vi "_TreeItem.Property.Set.Dictionary.Write.vi"(8 "error in (no error)":errorcluster, 11 "Dictionary":T1) -> (0 "error out":errorcluster, 3 "DictionaryProperty":refnum<k24>)   [LabVIEW 2017, in "Advanced System Definition.lvlib"]
uses:
  SysDef API/Advanced System Definition.lvlib
  _Types/Property.Dictionary.ctl
  NationalInstruments.VeriStand.SystemStorage
  _Types/Dictionary Item.ctl
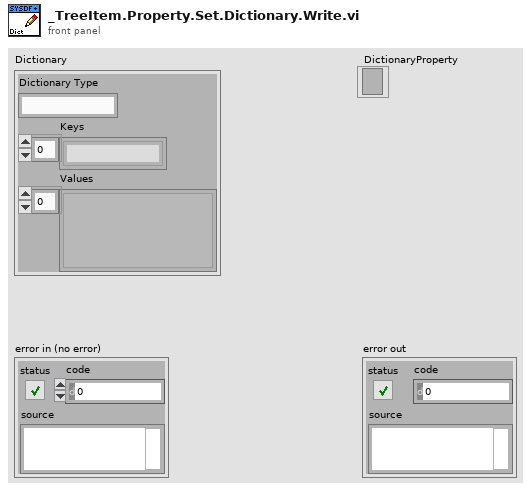
[diagram p1: front panel]
types:
  T1 = typedef "Advanced System Definition.lvlib/Property.Dictionary.ctl" = cluster{"Dictionary Type":string, "Keys":string[], "Values":variant[]}
  T2 = typedef "Advanced System Definition.lvlib/Dictionary Item.ctl" = cluster{"index":i32, "key":string, "value":variant}
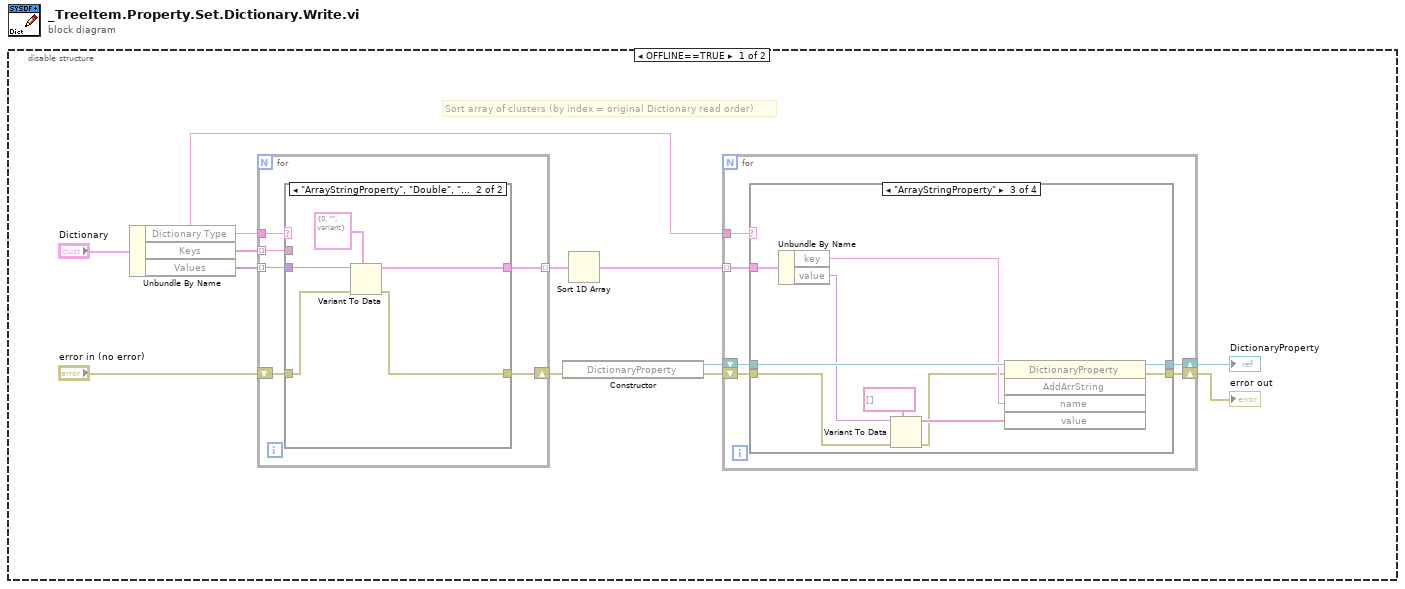
[diagram p0: block diagram]
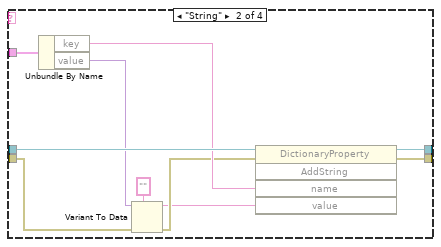
[diagram p3: hidden frame]
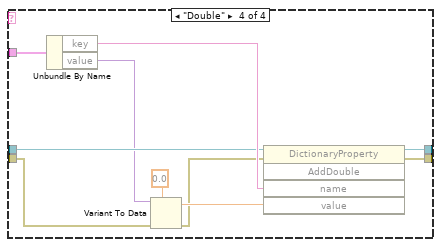
[diagram p4: hidden frame]
diagram:
  n1 = disable-structure shown="OFFLINE==TRUE" {
    frame condition #0 {
      # "Sort array of clusters (by index = original Dictionary read order)"
      n2 = Unbundle By Name("Dictionary") -> ("Dictionary Type"=w9:string, "Keys"=w10:string[], "Values"=w11:variant[])
      n3 = for {
        tunnel: w9 -> [w56]
        tunnel: w11 -> [w55] mode=indexing
        tunnel: w10 -> [w54] mode=indexing
        shift-right: [w52] -> w4
        shift-left: "error in (no error)" -> [w53]
        tunnel: [w51] -> w6 mode=indexing
        n4 = case shown="\"ArrayStringProperty\", \"Double\", \"String\"" w56 {
          tunnel: w54 -> [_ _]
          tunnel: w55 -> [_ w62]
          tunnel: w53 -> [w57 w61]
          tunnel: [w57 w60] -> w52
          tunnel: [_ w59] -> w51
          frame Default {
          }
          frame "ArrayStringProperty", "Double", "String" {
            n5 = Variant To Data(error in=w61, type=T2 {"index"=0, "key"="", "value"=variant} ("Dictionary Item"), Variant=w62) -> (data=w59:T2, error out=w60:errorcluster)
          }
        }
      }
      n6 = constructor class="DictionaryProperty"(error in=w4) -> (reference out=w2:refnum<k24>, error out=w3:errorcluster)  [unwired: 2 in, 1 out]
      n7 = Sort 1D Array(array=w6) -> (sorted array=w5:T2[])
      n8 = for {
        shift-right: [w17] -> w8
        shift-left: w2 -> [w18]
        tunnel: w9 -> [w16]
        shift-right: [w14] -> w7
        shift-left: w3 -> [w15]
        tunnel: w5 -> [w13] mode=indexing
        n9 = case shown="\"ArrayStringProperty\"" w16 {
          tunnel: w18 -> [w20 w30 w40 w46]
          tunnel: [w20 w29 w39 w50] -> w17
          tunnel: w15 -> [w19 w23 w32 w42]
          tunnel: [w19 w28 w38 w49] -> w14
          tunnel: w13 -> [_ w27 w36 w47]
          frame Default {
          }
          frame "String" {
            n10 = Unbundle By Name(w27) -> ("key"=w26:string, "value"=w24:variant)
            n11 = Variant To Data(error in=w23, type="", Variant=w24) -> (data=w21:string, error out=w22:errorcluster)
            n12 = invoke class="DictionaryProperty" method="AddString"(reference=w30, error in=w22, "name"=w26, "value"=w21) -> (reference out=w29:refnum<k24>, error out=w28:errorcluster)  [unwired: 1 in, 3 out]
          }
          frame "ArrayStringProperty" {
            n13 = Unbundle By Name(w36) -> ("key"=w37:string, "value"=w34:variant)
            n14 = Variant To Data(error in=w32, type=string[] [], Variant=w34) -> (data=w33:string[], error out=w31:errorcluster)
            n15 = invoke class="DictionaryProperty" method="AddArrString"(reference=w40, error in=w31, "name"=w37, "value"=w33) -> (reference out=w39:refnum<k24>, error out=w38:errorcluster)  [unwired: 1 in, 3 out]
          }
          frame "Double" {
            n16 = Unbundle By Name(w47) -> ("key"=w48:string, "value"=w44:variant)
            n17 = Variant To Data(error in=w42, type=0.0, Variant=w44) -> (data=w43:dbl, error out=w41:errorcluster)
            n18 = invoke class="DictionaryProperty" method="AddDouble"(reference=w46, error in=w41, "name"=w48, "value"=w43) -> (reference out=w50:refnum<k24>, error out=w49:errorcluster)  [unwired: 1 in, 3 out]
          }
        }
      }
      "error out" <- w7
      "DictionaryProperty" <- w8
    }
    frame condition #1 (active) {
    }
  }
